vi "GetWindowRect.vi"(8 "错误输入（无错误）":errorcluster, 11 "WindowHandle":u32) -> (0 "错误输出":errorcluster, 2 "Rect":T1, 3 "Result":bool)   [LabVIEW 2018, in "Win32API.lvlib"]
uses:
  Win32API.lvlib
  user32.dll
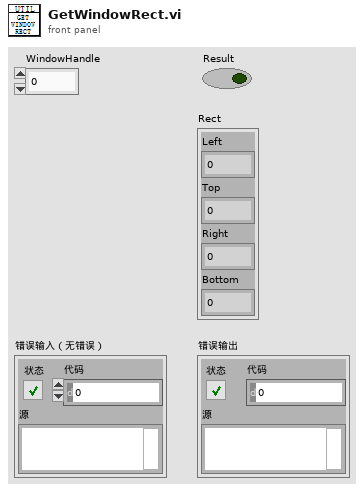
[diagram p1: front panel]
types:
  T1 = cluster{"Left":i32, "Top":i32, "Right":i32, "Bottom":i32}
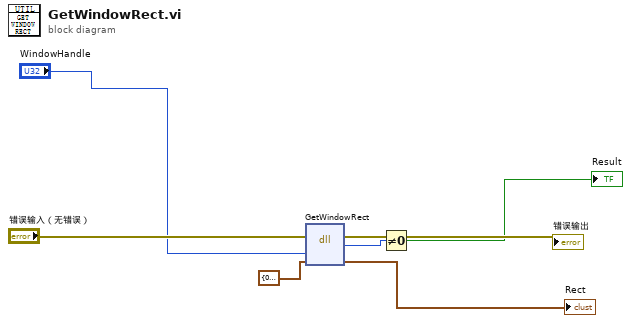
[diagram p0: block diagram]
diagram:
  n1 = dll-call lib="user32.dll" fn="GetWindowRect"(error in="错误输入（无错误）", "Handle"="WindowHandle", "Rect"=T1 {"Left"=0, "Top"=0, "Right"=0, "Bottom"=0} ("前面板窗口:窗口边界")) -> (error out=→"错误输出":errorcluster, "Result"=w2:i32, "Rect"=→"Rect":T1)  [unwired: 3 in, 1 out]
  n2 = Not Equal To 0?(x=w2) -> (x != 0?=→"Result":bool)
